vi "AC2250 Measurement Channel.vi"(7 "Term Char":enum16{"Cr/Lf"}(ring), 8 "ErrIn":errorcluster, 10 "Reference":bool, 11 "VISA Resource Name In":refnum<visa-resource-name>) -> (0 "ErrOut":errorcluster, 2 "Return Count":i32, 3 "VISA Resource Name Out":refnum<visa-resource-name>)   [LabVIEW 2013]
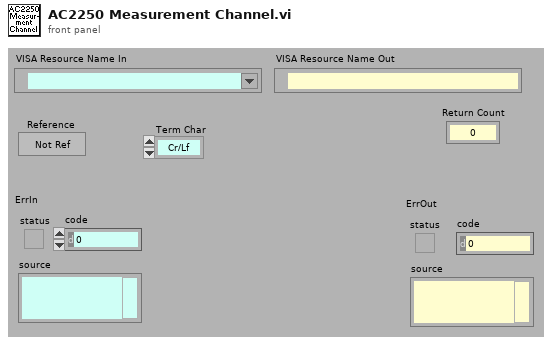
[diagram p1: front panel]
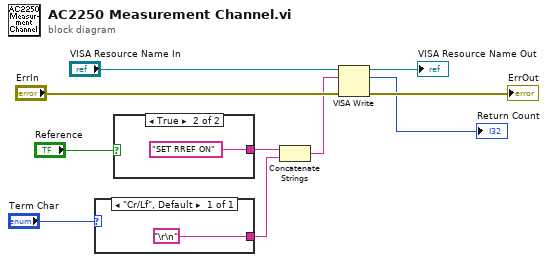
[diagram p0: block diagram]
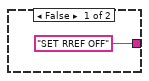
[diagram p2: hidden frame]
diagram:
  n1 = case shown="\"Cr/Lf\", Default" "Term Char" {
    tunnel: ["\r\n"] -> w4
    frame "Cr/Lf", Default {
    }
  }
  n2 = case shown="True" "Reference" {
    tunnel: ["SET RREF OFF" "SET RREF ON"] -> w6
    frame False {
    }
    frame True {
    }
  }
  n3 = Concatenate Strings(w6, w4) -> (w3:string)
  n4 = VISA Write(VISA resource name="VISA Resource Name In", write buffer=w3, error in (no error)="ErrIn") -> (VISA resource name out=→"VISA Resource Name Out":refnum<visa-resource-name>, return count=→"Return Count":u32, error out=→"ErrOut":errorcluster)
